vi "FGV - Acquisition Status.vi"(7 "Actions":T2=enum."Clear", 8 "error in (no error)":errorcluster, 11 "Action":T1) -> (0 "error out":errorcluster, 3 "Action [Out]":T1)   [LabVIEW 2017]
uses:
  Controls/FGV Actions.ctl
  Controls/Thorlabs Acq Status.ctl
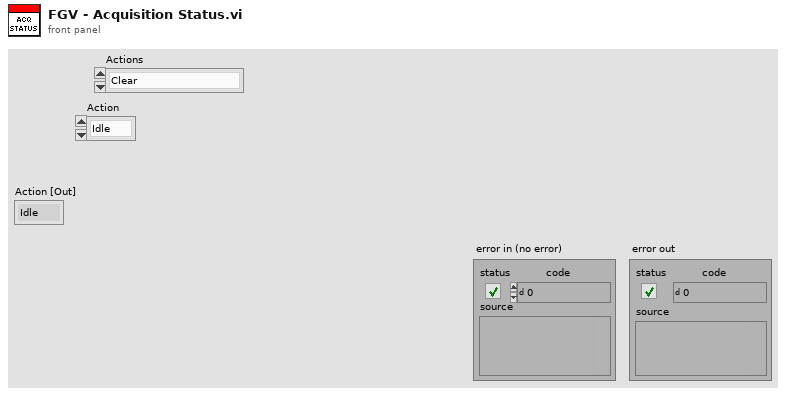
[diagram p1: front panel]
types:
  T1 = typedef "Thorlabs Acq Status.ctl" = enum16{"Idle", "Image", "Translate"}
  T2 = typedef "FGV Actions.ctl" = enum16{"Init", "Set", "Get", "Clear"}
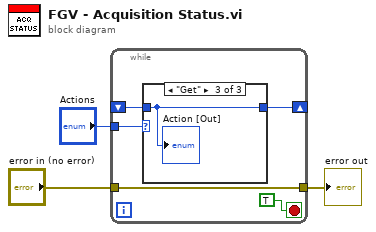
[diagram p0: block diagram]
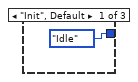
[diagram p2: hidden frame]
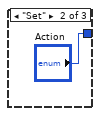
[diagram p3: hidden frame]
diagram:
  n1 = while {
    tunnel: "Actions" -> [w8]
    shift-right: [w6] -> _
    shift-left: _ -> [w5]
    tunnel: "error in (no error)" -> [w4]
    tunnel: [w4] -> w1
    stop <- TRUE stop-if-true
    n2 = case shown="\"Get\"" w8 {
      tunnel: [Thorlabs_Acq_Status."Idle" "Action" w11] -> w6
      tunnel: w5 -> [_ _ w11]
      frame "Init", Default {
      }
      frame "Set" {
      }
      frame "Get" {
        "Action [Out]" <- w11
      }
    }
  }
  "error out" <- w1
